vi "Excel Set Cell Color and Border.vi"(0 "report in":refnum<class "NI_report.lvclass">, 1 "inside border":T1={"on/off"=FALSE, "weight"=2, "color"=0} {"weight" items=["xlHairline"=1, "xlMedium"=-4138, "xlThick"=4, "xlThin"=2]}, 2 "outside border":T1={"on/off"=FALSE, "weight"=2, "color"=0} {"weight" items=["xlHairline"=1, "xlMedium"=-4138, "xlThick"=4, "xlThin"=2]}, 5 "background color (w)":u32(colorbox)=16777215, 7 "start (-1, -1)":cluster{"row":i32, "column":i32}={"row"=-1, "column"=-1}, 9 "end (-1, -1)":cluster{"row":i32, "column":i32}={"row"=-1, "column"=-1}, 11 "error in (no error)":errorcluster, 12 "name (\"\")":string) -> (4 "report out":refnum<class "NI_report.lvclass">, 15 "error out":errorcluster)   [LabVIEW 2017, in "NI_Excel.lvclass"]
doc: "Sets the borders and background color of the cells specified by the <B>start</B> and <B>end</B> clusters or by a named range."
uses:
  <vilib>/Utility/NIReport.llb/Excel/NI_Excel.lvclass
  <vilib>/addons/_office/NI_ReportGenerationToolkit.lvlib
  <vilib>/Utility/NIReport.llb/NI_ReportGenerationCore.lvlib
  C:/Program Files (x86)/National Instruments/LabVIEW 2017/vi.lib/Utility/NIReport.llb/NI_report.lvclass
  <vilib>/Utility/NIReport.llb/NI_report.lvclass
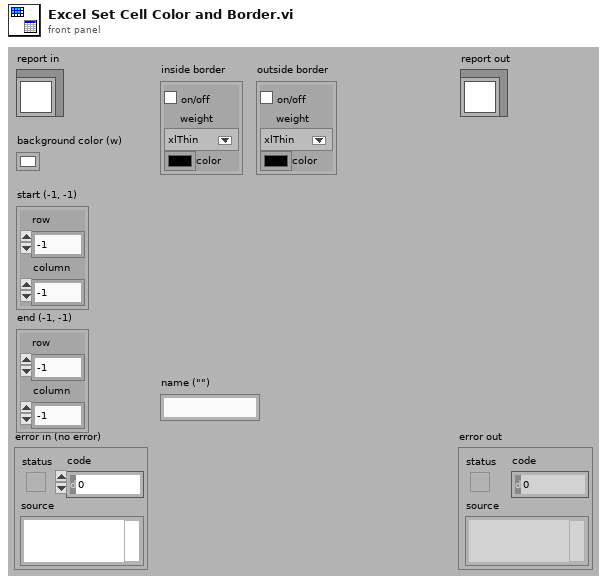
[diagram p1: front panel]
types:
  T1 = cluster{"on/off":bool, "weight":i32, "color":u32}
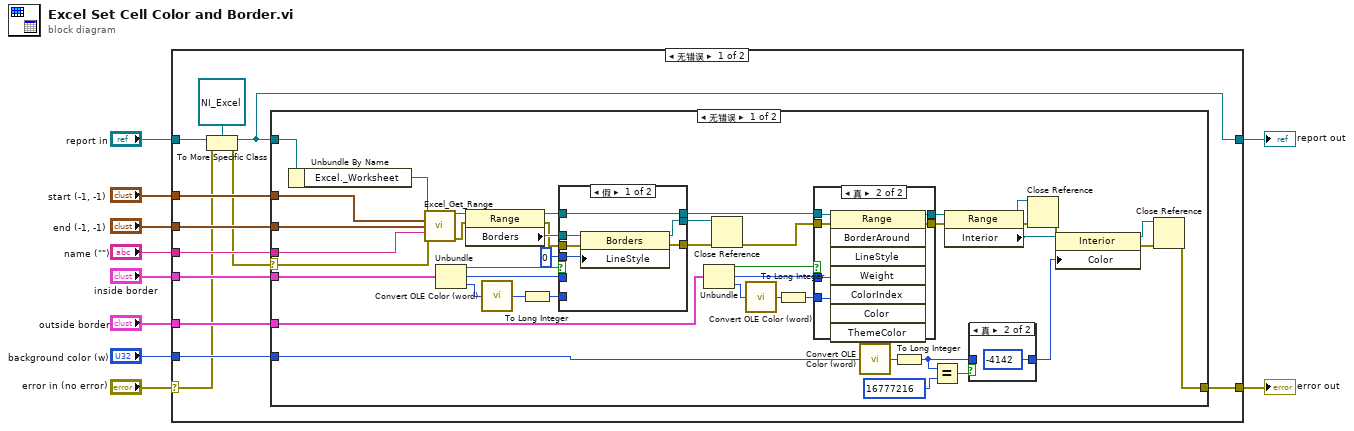
[diagram p0: block diagram]
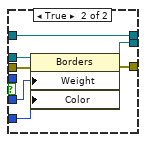
[diagram p4: hidden frame]
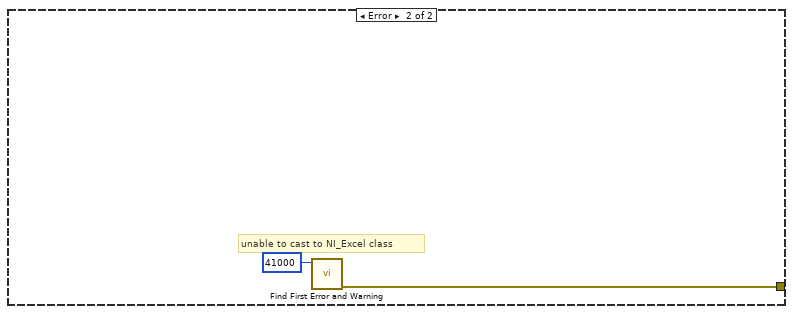
[diagram p5: hidden frame]
diagram:
  n1 = case shown="无错误" "error in (no error)" {
    selector: "error in (no error)" -> [w11 w92]
    tunnel: [w16 w92] -> w9
    tunnel: [w13 w91] -> w7
    tunnel: "report in" -> [w14 w91]
    tunnel: "start (-1, -1)" -> [w22 _]
    tunnel: "end (-1, -1)" -> [w21 _]
    tunnel: "name (\"\")" -> [w20 _]
    tunnel: "inside border" -> [w19 _]
    tunnel: "outside border" -> [w18 _]
    tunnel: "background color (w)" -> [w17 _]
    frame No Error {
      n2 = To More Specific Class(target class=refnum<class "NI_Excel.lvclass"> refnum ("report in"), reference=w14, error in=w11) -> (specific class reference=w13:refnum<class "NI_Excel.lvclass">, error out=w12:errorcluster)
      n3 = case shown="无错误" w12 {
        selector: w12 -> [w27 _]
        tunnel: w13 -> [w36 _]
        tunnel: w22 -> [w35 _]
        tunnel: w21 -> [w34 _]
        tunnel: w20 -> [w33 _]
        tunnel: w19 -> [w32 _]
        tunnel: w18 -> [w31 _]
        tunnel: w17 -> [w30 _]
        tunnel: [w29 w89] -> w16
        frame No Error {
          n4 = Unbundle By Name(w36) -> ("Excel._Worksheet"=w28:refnum<k7>)
          n5 = call <vilib>:"Excel_Get_Range.vi"("Excel._Worksheet"=w28, "start"=w35, "end"=w34, "name"=w33, "error in (no error)"=w27) -> ("Range"=w61:refnum<k7>, "error out"=w62:errorcluster)  [unwired: 5 in, 4 out]
          n6 = Unbundle(w32) -> ("on/off"=w55:bool, "weight"=w53:i32, "color"=w52:u32)
          n7 = property class="Range"(reference=w61, error in=w62) -> (reference out=w56:refnum<k7>, error out=w46:errorcluster, "Borders"=w54:refnum<k7>)
          n8 = call <vilib>:"Convert OLE Color (word).vi"("color in"=w52) -> ("color out"=w38:u32)
          n9 = To Long Integer(number=w38) -> (32bit integer=w63:i32)
          n10 = case shown="假" w55 {
            tunnel: w63 -> [_ w88]
            tunnel: [w77 w87] -> w44
            tunnel: [w79 w86] -> w45
            tunnel: w46 -> [w80 w85]
            tunnel: w53 -> [_ w84]
            tunnel: w54 -> [w78 w83]
            tunnel: w56 -> [w81 w82]
            tunnel: [w81 w82] -> w57
            tunnel: 0 -> [w76 _]
            frame False {
              n11 = property class="Borders"(reference=w78, error in=w80, "LineStyle"=w76) -> (reference out=w77:refnum<k7>, error out=w79:errorcluster)
            }
            frame True {
              n12 = property class="Borders"(reference=w83, error in=w85, "Weight"=w84, "Color"=w88) -> (reference out=w87:refnum<k7>, error out=w86:errorcluster)
            }
          }
          n13 = Unbundle(w31) -> ("on/off"=w60:bool, "weight"=w59:i32, "color"=w58:u32)
          n14 = Close Reference(reference=w44, error in (no error)=w45) -> (error out=w48:errorcluster)
          n15 = call <vilib>:"Convert OLE Color (word).vi"("color in"=w58) -> ("color out"=w51:u32)
          n16 = To Long Integer(number=w51) -> (32bit integer=w64:i32)
          n17 = case shown="真" w60 {
            tunnel: w48 -> [w68 w75]
            tunnel: [w68 w74] -> w49
            tunnel: [w69 w73] -> w50
            tunnel: w64 -> [_ w72]
            tunnel: w57 -> [w69 w71]
            tunnel: w59 -> [_ w70]
            frame False {
            }
            frame True {
              n18 = invoke class="Range" method="BorderAround"(reference=w71, error in=w75, "Weight"=w70, "Color"=w72) -> (reference out=w73:refnum<k7>, error out=w74:errorcluster)  [unwired: 4 in, 6 out]
            }
          }
          n19 = call <vilib>:"Convert OLE Color (word).vi"("color in"=w30) -> ("color out"=w37:u32)
          n20 = To Long Integer(number=w37) -> (32bit integer=w24:i32)
          n21 = Equal?(x=w24, y=16777216) -> (x = y?=w25:bool)
          n22 = property class="Range"(reference=w50, error in=w49) -> (reference out=w40:refnum<k7>, error out=w42:errorcluster, "Interior"=w47:refnum<k7>)
          n23 = case shown="真" w25 {
            tunnel: w24 -> [w66 _]
            tunnel: [w66 -4142] -> w23
            frame False {
            }
            frame True {
            }
          }
          n24 = Close Reference(reference=w40, error in (no error)=w42) -> (error out=w41:errorcluster)
          n25 = property class="Interior"(reference=w47, error in=w41, "Color"=w23) -> (reference out=w39:refnum<k7>, error out=w43:errorcluster)
          n26 = Close Reference(reference=w39, error in (no error)=w43) -> (error out=w29:errorcluster)
        }
        frame Error {
          # "unable to cast to NI_Excel class"
          n27 = call <vilib>:"Find First Error and Warning.vi"("error code"=41000) -> ("error out"=w89:errorcluster)  [unwired: 2 in, 4 out]
        }
      }
    }
    frame Error {
    }
  }
  "error out" <- w9
  "report out" <- w7
